vi "LEDC SWIR 1931 Init_2015LED.vi"(0 "LEDAD Port":refnum<visa-resource-name>="COM7", 1 "Wavelength":string, 5 "Light Meter Port":refnum<visa-resource-name>="COM4", 11 "error in (no error)":errorcluster, 12 "2015 LED":bool) -> (3 "In Progress":bool, 4 "LEDAD Port out":refnum<visa-resource-name>, 6 "Light Meter Port out":refnum<visa-resource-name>, 14 "Done":bool, 15 "error out":errorcluster)   [LabVIEW 2010]
panel:
  # "nm"
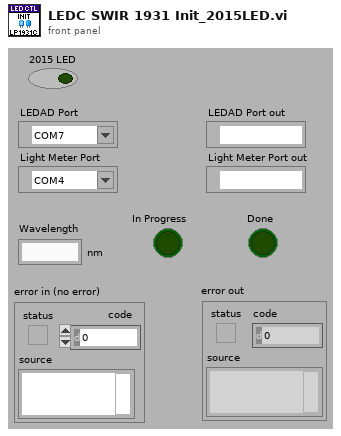
[diagram p1: front panel]
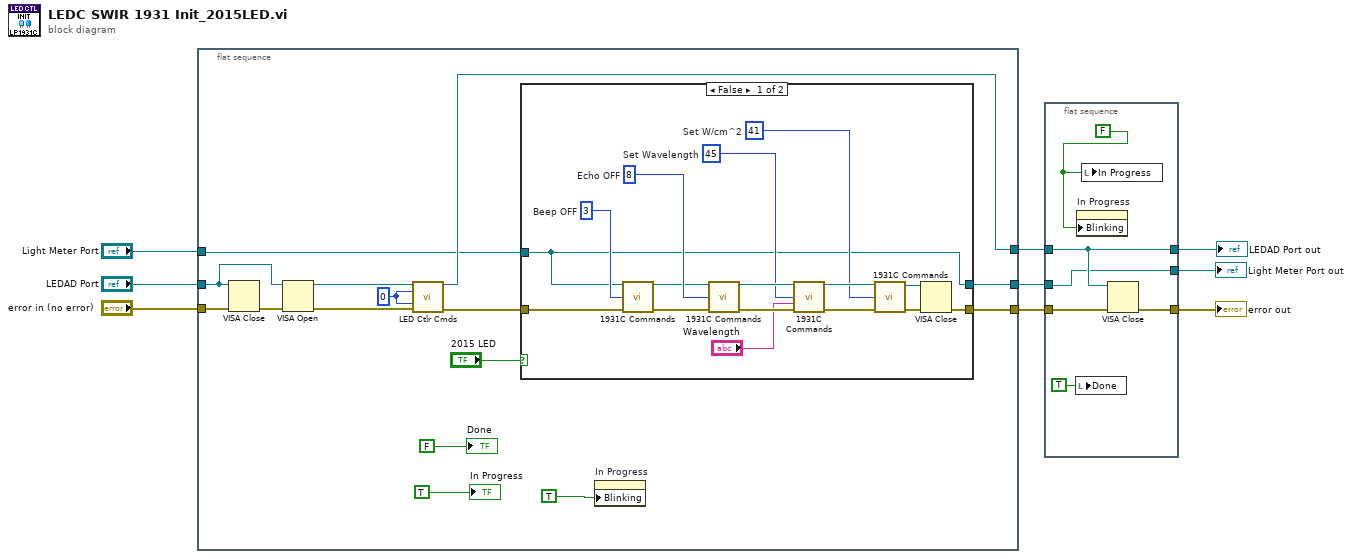
[diagram p0: block diagram]
diagram:
  n1 = flat-sequence {
    tunnel: "error in (no error)" -> [w24]
    tunnel: "LEDAD Port" -> [w22]
    tunnel: "Light Meter Port" -> [w14]
    tunnel: [w18] -> w2
    tunnel: [w17] -> w3
    tunnel: [w16] -> w1
    frame #0 {
      w15 = 0
      n2 = VISA Close(VISA resource name=w22, error in (no error)=w24) -> (error out=w23:errorcluster)
      n3 = VISA Open(error in (no error)=w23, VISA resource name=w22) -> (VISA resource name=w12:refnum<visa-resource-name>, error out=w11:errorcluster)  [unwired: 3 in]
      n4 = call "LED Ctlr Cmds.vi"("VISA session"=w12, "Intensity"=w15, "Enable"=w15, "error in (no error)"=w11) -> ("VISA session out"=w16:refnum<visa-resource-name>, "error out"=w13:errorcluster)  [unwired: 7 in, 3 out]
      n5 = case shown="False" "2015 LED" {
        tunnel: [w25 w41] -> w18
        tunnel: [w27 w42] -> w17
        tunnel: w14 -> [w25 w41]
        tunnel: w13 -> [w32 w42]
        frame False {
          w29 = 3  # Beep OFF
          w34 = 41  # Set W/cm^2
          w37 = 45  # Set Wavelength
          w40 = 8  # Echo OFF
          n6 = call "1931C Commands.vi"("Instrument Resource Name"=w25, "Command"=w29, "error in (no error)"=w32) -> ("VISA resource name out"=w31:refnum<visa-resource-name>, "error out"=w30:errorcluster)  [unwired: 8 in, 3 out]
          n7 = call "1931C Commands.vi"("Instrument Resource Name"=w31, "Command"=w40, "error in (no error)"=w30) -> ("VISA resource name out"=w38:refnum<visa-resource-name>, "error out"=w39:errorcluster)  [unwired: 8 in, 3 out]
          n8 = call "1931C Commands.vi"("Instrument Resource Name"=w38, "Command"=w37, "Wavelength"="Wavelength", "error in (no error)"=w39) -> ("VISA resource name out"=w35:refnum<visa-resource-name>, "error out"=w36:errorcluster)  [unwired: 7 in, 3 out]
          n9 = call "1931C Commands.vi"("Instrument Resource Name"=w35, "Command"=w34, "error in (no error)"=w36) -> ("VISA resource name out"=w26:refnum<visa-resource-name>, "error out"=w28:errorcluster)  [unwired: 8 in, 3 out]
          n10 = VISA Close(VISA resource name=w26, error in (no error)=w28) -> (error out=w27:errorcluster)
        }
        frame True {
        }
      }
      n11 = property on="In Progress" class="Bool (strict)"("Blinking"=TRUE) -> ()  [unwired: 2 in, 2 out]
      "Done" <- FALSE
      "In Progress" <- TRUE
    }
  }
  n12 = flat-sequence {
    tunnel: w2 -> [w45]
    tunnel: w3 -> [w43]
    tunnel: [w46] -> w4
    tunnel: w1 -> [w46]
    tunnel: [w45] -> w5
    tunnel: [w44] -> w6
    frame #0 {
      w48 = FALSE
      n13 = local write "Done"(TRUE) -> ()
      n14 = property on="In Progress" class="Bool (strict)"("Blinking"=w48) -> ()  [unwired: 2 in, 2 out]
      n15 = local write "In Progress"(w48) -> ()
      n16 = VISA Close(VISA resource name=w46, error in (no error)=w43) -> (error out=w44:errorcluster)
    }
  }
  "LEDAD Port out" <- w4
  "Light Meter Port out" <- w5
  "error out" <- w6
